vi "Update Channel Data.vi"(8 "error in (no error)":errorcluster, 9 "index":i32, 10 "channel data":cluster{"Y":dbl[], "channel attributes":variant}, 11 "Y (N Ch) in":refnum<class "Y (N Ch).lvclass">) -> (0 "error out":errorcluster, 3 "Y (N Ch) out":refnum<class "Y (N Ch).lvclass">)   [LabVIEW 2017, in "Y (N Ch).lvclass"]
uses:
  <vilib>/addons/_NISVFA/_Shared subVIs/Data Objects/Y (DBL)/Y (N Ch).lvclass
  <vilib>/addons/_NISVFA/_Shared subVIs/Data Objects/Y (DBL)/Y (N Ch).lvclass/Y (N Ch).ctl
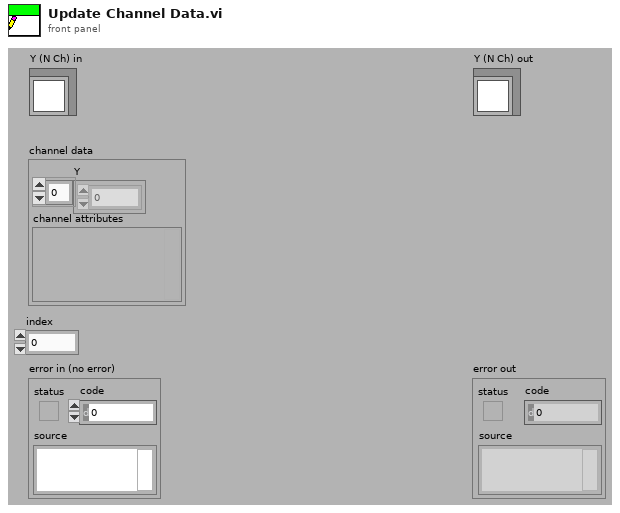
[diagram p1: front panel]
types:
  T1 = cluster{"Y":dbl[], "channel attributes":variant}[]
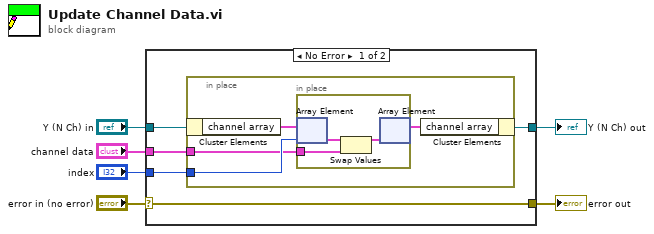
[diagram p0: block diagram]
diagram:
  n1 = case shown="No Error" "error in (no error)" {
    selector: "error in (no error)" -> [w11 w19]
    tunnel: [w11 w19] -> w5
    tunnel: [w9 w20] -> w3
    tunnel: "Y (N Ch) in" -> [w10 w20]
    tunnel: "channel data" -> [w7 _]
    tunnel: "index" -> [w8 _]
    frame No Error {
      n2 = in-place {
        in-place-border: w8 -> [w14]
        in-place-border: w7 -> [w12]
        n3 = in-place-cluster #1(w10) -> ("channel array"=w15:T1)
        n4 = in-place {
          in-place-border: w12 -> [w16]
          n5 = in-place-array #2(w15, w14) -> (w18:cluster{"Y":dbl[], "channel attributes":variant})
          n6 = Swap Values(12:w18, 14:w16) -> (1:w17:cluster{"Y":dbl[], "channel attributes":variant})  [unwired: 1 in, 1 out]
          n7 = in-place-array #2(w17) -> (w13:T1)  [unwired: 1 out]
        }
        n8 = in-place-cluster #1("channel array"=w13) -> (w9:refnum<class "Y (N Ch).lvclass">)
      }
    }
    frame Error {
    }
  }
  "error out" <- w5
  "Y (N Ch) out" <- w3
